vi "CreateBoundingBox.vi"(8 "error in (no error)":errorcluster, 11 "class data in":refnum<class "BoundingBox.lvclass">) -> (0 "error out":errorcluster, 3 "class data out":refnum<class "BoundingBox.lvclass">)   [LabVIEW 2010, in "Labricks.lvlib" / "BoundingBox.lvclass"]
uses:
  BoundingBox.lvclass
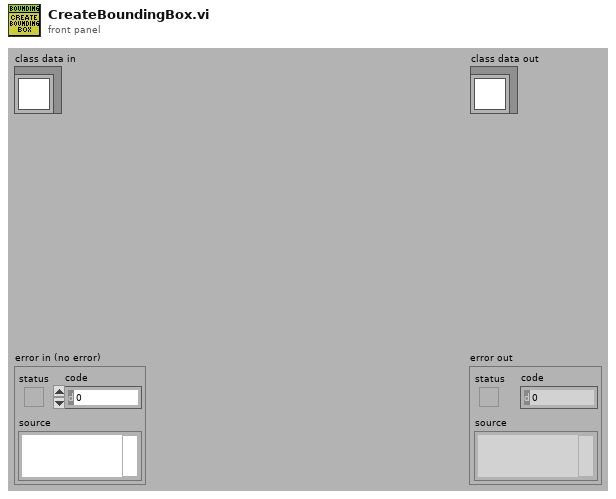
[diagram p1: front panel]
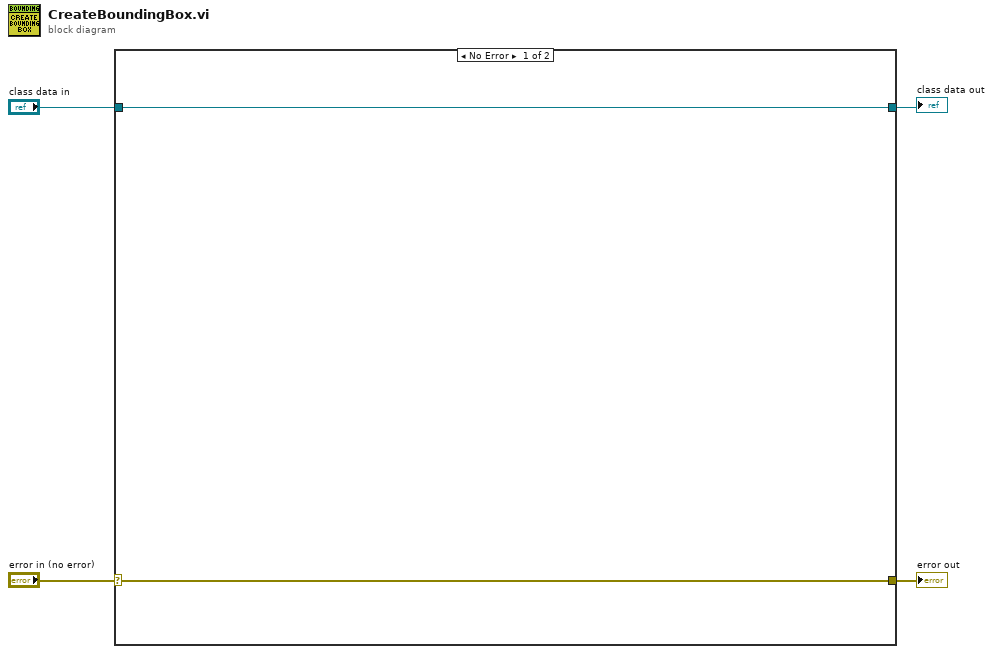
[diagram p0: block diagram]
diagram:
  n1 = case shown="No Error" "error in (no error)" {
    selector: "error in (no error)" -> [w6 w8]
    tunnel: [w6 w8] -> w3
    tunnel: "class data in" -> [w5 w7]
    tunnel: [w5 w7] -> w1
    frame No Error {
    }
    frame Error {
    }
  }
  "error out" <- w3
  "class data out" <- w1
